vi "CT_PSExpandArray.vi"(0 "Array of Power Supply Delay and Enable":cluster{"PS Delay":dbl, "PS Enable":bool}[](array[cluster])) -> (1 "PS1 Cluster":cluster{"PS Delay":dbl, "PS Enable":bool}, 2 "PS6 Cluster":cluster{"PS Delay":dbl, "PS Enable":bool}, 3 "PS2 Cluster":cluster{"PS Delay":dbl, "PS Enable":bool}, 4 "PS3 Cluster":cluster{"PS Delay":dbl, "PS Enable":bool}, 5 "PS4 Cluster":cluster{"PS Delay":dbl, "PS Enable":bool}, 6 "PS5 Cluster":cluster{"PS Delay":dbl, "PS Enable":bool})   [LabVIEW 2016]
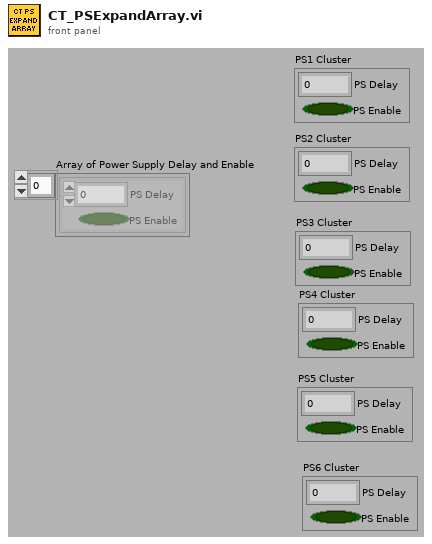
[diagram p1: front panel]
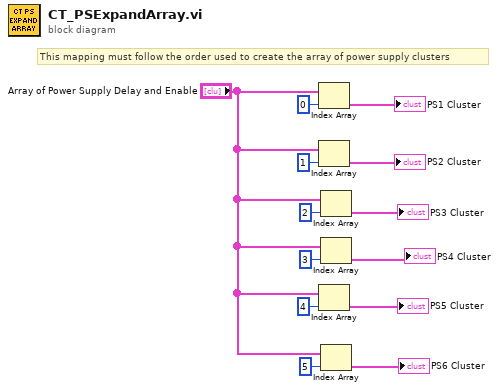
[diagram p0: block diagram]
diagram:
  # "This mapping must follow the order used to create the array of power supply clusters"
  n1 = Index Array(array="Array of Power Supply Delay and Enable", index=0) -> (element=→"PS1 Cluster":cluster{"PS Delay":dbl, "PS Enable":bool})
  n2 = Index Array(array="Array of Power Supply Delay and Enable", index=1) -> (element=→"PS2 Cluster":cluster{"PS Delay":dbl, "PS Enable":bool})
  n3 = Index Array(array="Array of Power Supply Delay and Enable", index=4) -> (element=→"PS5 Cluster":cluster{"PS Delay":dbl, "PS Enable":bool})
  n4 = Index Array(array="Array of Power Supply Delay and Enable", index=2) -> (element=→"PS3 Cluster":cluster{"PS Delay":dbl, "PS Enable":bool})
  n5 = Index Array(array="Array of Power Supply Delay and Enable", index=3) -> (element=→"PS4 Cluster":cluster{"PS Delay":dbl, "PS Enable":bool})
  n6 = Index Array(array="Array of Power Supply Delay and Enable", index=5) -> (element=→"PS6 Cluster":cluster{"PS Delay":dbl, "PS Enable":bool})
